vi "BooleanLatchUpdate.vi"(8 "error in":errorcluster, 10 "Control Value in":variant, 11 "Control in":refnum<vi>) -> (0 "error out":errorcluster, 2 "Control Value out":variant)   [LabVIEW 2025, in "UI_Library.lvlib" / "UI_Library.lvclass"]
uses:
  UI_Library.lvclass
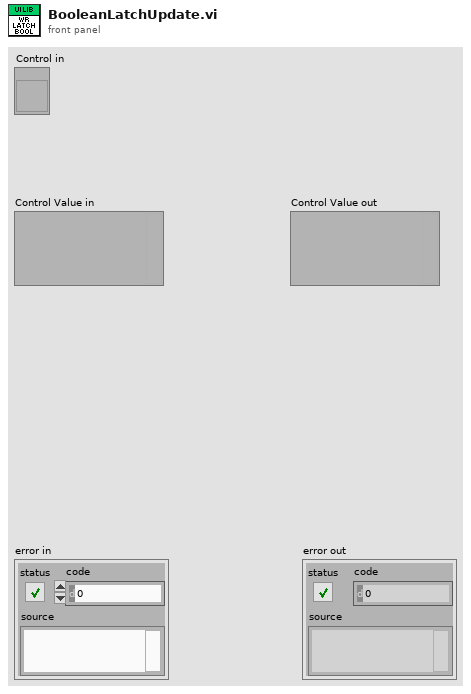
[diagram p1: front panel]
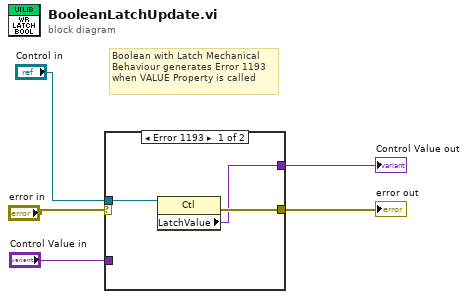
[diagram p0: block diagram]
diagram:
  # "Boolean with Latch Mechanical\nBehaviour generates Error 1193 \nwhen VALUE Property is called"
  n1 = case shown="Error 1193" "error in" {
    selector: "error in" -> [_ w9]
    tunnel: "Control in" -> [w8 _]
    tunnel: [w7 w9] -> w2
    tunnel: [w6 w10] -> w4
    tunnel: "Control Value in" -> [_ w10]
    frame #0 {
      n2 = property on="Property Node" class="Ctl"(reference=w8) -> (error out=w7:errorcluster, "LatchValue"=w6:variant)  [unwired: 1 in, 1 out]
    }
    frame #1 {
    }
  }
  "Control Value out" <- w4
  "error out" <- w2
